vi "Transfer Configuration.Get Byte Order.vi"(11 "Transfer Configuration in":refnum<class "Transfer Configuration.lvclass">) -> (2 "byte order":T1, 3 "Transfer Configuration out":refnum<class "Transfer Configuration.lvclass">)   [LabVIEW 2017, in "DSF Core.lvlib" / "Transfer Configuration.lvclass"]
uses:
  Transfer Configuration.lvclass
  DSF Configuration API/Public/Controls/DSF Byte Order.ctl
  Transfer Configuration.lvclass/Transfer Configuration.ctl
  DSF Core.lvlib
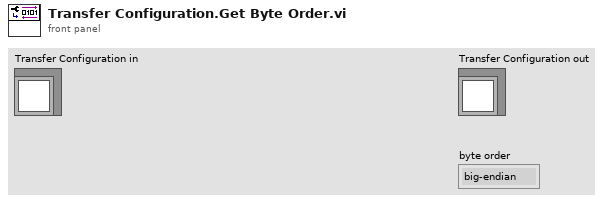
[diagram p1: front panel]
types:
  T1 = typedef "DSF Core.lvlib/DSF Byte Order.ctl" = enum8{"big-endian", "little-endian"}
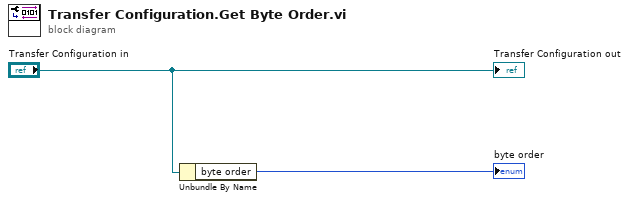
[diagram p0: block diagram]
diagram:
  n1 = Unbundle By Name("Transfer Configuration in") -> ("byte order"=→"byte order":T1)
  "Transfer Configuration out" <- "Transfer Configuration in"
